vi "Clean Up Actor.vi"(8 "error in (no error)":errorcluster, 11 "Terminal Timeout in":refnum<class "Terminal Timeout.lvclass">) -> (0 "error out":errorcluster, 3 "Terminal Timeout out":refnum<class "Terminal Timeout.lvclass">)   [LabVIEW 2016, in "CLD Exam - ATM.lvlib" / "Terminal Timeout.lvclass"]
uses:
  Terminal Timeout.lvclass
  D:/Repos/Stream/software/Mediator/Classes/Mediated Actor/Mediated Actor.lvclass
  Mediator/Classes/Message Broker Interface/Message Broker Interface.lvclass
  Mediator/Classes/Mediated Synchronous Actor/Mediated Synchronous Actor.lvclass
  Mediator/Classes/Mediated Actor/Mediated Actor.lvclass
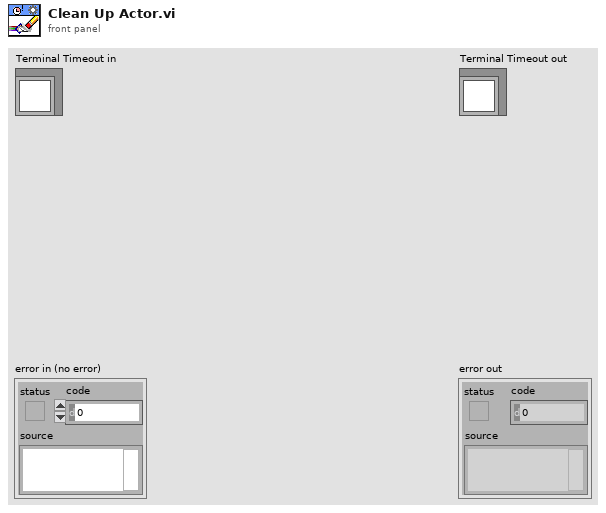
[diagram p1: front panel]
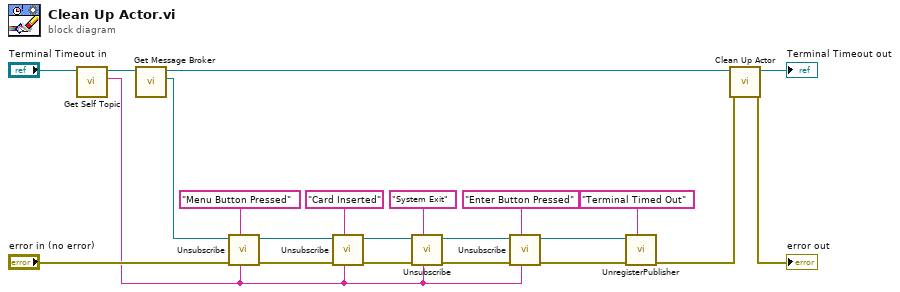
[diagram p0: block diagram]
diagram:
  n1 = call "Get Self Topic.vi"("Mediated Actor in"="Terminal Timeout in") -> ("Topic.Self"=w7:string, "Mediated Actor out"=w18:refnum<class "Terminal Timeout.lvclass">)  [unwired: 9 in]
  n2 = call "Get Message Broker.vi"("Mediated Actor in"=w18) -> ("Message Broker"=w15:refnum<class "Message Broker Interface.lvclass">, "Mediated Actor out"=w16:refnum<class "Terminal Timeout.lvclass">)  [unwired: 9 in]
  n3 = call-dynamic "Unsubscribe.vi"("Subscriber Name"=w7, "Topic Name"="Menu Button Pressed", "error in (no error)"="error in (no error)", "Message Broker Interface in"=w15) -> ("error out"=w1:errorcluster, "Message Broker Interface out"=w2:refnum<class "Message Broker Interface.lvclass">)  [unwired: 6 in]
  n4 = call-dynamic "Unsubscribe.vi"("Subscriber Name"=w7, "Topic Name"="Card Inserted", "error in (no error)"=w1, "Message Broker Interface in"=w2) -> ("error out"=w12:errorcluster, "Message Broker Interface out"=w11:refnum<class "Message Broker Interface.lvclass">)  [unwired: 6 in]
  n5 = call-dynamic "Unsubscribe.vi"("Subscriber Name"=w7, "Topic Name"="System Exit", "error in (no error)"=w12, "Message Broker Interface in"=w11) -> ("error out"=w9:errorcluster, "Message Broker Interface out"=w8:refnum<class "Message Broker Interface.lvclass">)  [unwired: 6 in]
  n6 = call-dynamic "Unsubscribe.vi"("Subscriber Name"=w7, "Topic Name"="Enter Button Pressed", "error in (no error)"=w9, "Message Broker Interface in"=w8) -> ("error out"=w5:errorcluster, "Message Broker Interface out"=w4:refnum<class "Message Broker Interface.lvclass">)  [unwired: 6 in]
  n7 = call-dynamic "UnregisterPublisher.vi"("Topic Name"="Terminal Timed Out", "error in (no error)"=w5, "Message Broker Interface in"=w4) -> ("error out"=w3:errorcluster)  [unwired: 7 in, 1 out]
  n8 = call-parent "Clean Up Actor.vi"("error in (no error)"=w3, "Mediated Actor in"=w16) -> ("error out"=→"error out":errorcluster, "Mediated Actor out"=→"Terminal Timeout out":refnum<class "Terminal Timeout.lvclass">)  [unwired: 8 in]
